vi "interface alive.vi"(8 "error in (no error)":errorcluster, 11 "output_actor in":refnum<class "Output Actor.lvclass">) -> (0 "error out":errorcluster, 2 "alive":bool, 3 "output_actor out":refnum<class "Output Actor.lvclass">)   [LabVIEW 2015, in "Output Actor.lvclass"]
uses:
  Output Actor.lvclass
  Output Actor.lvclass/Output Actor.ctl
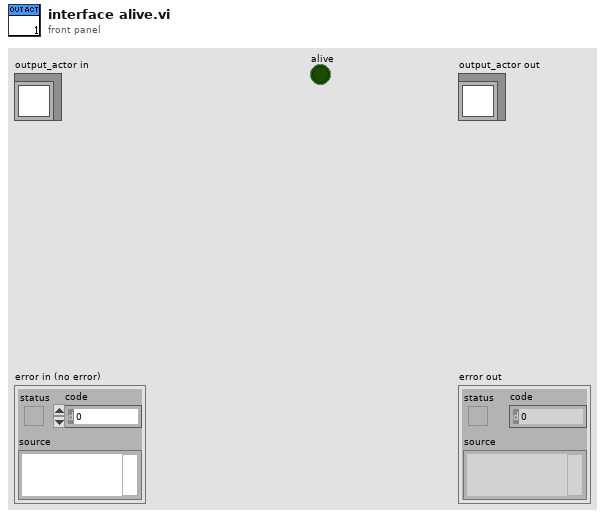
[diagram p1: front panel]
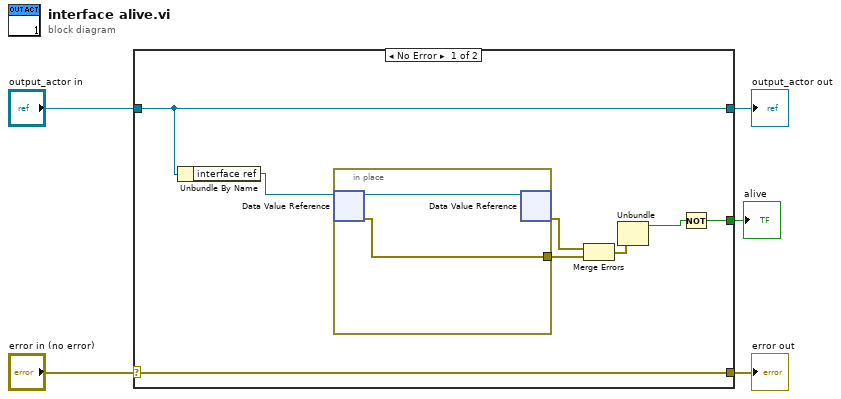
[diagram p0: block diagram]
diagram:
  n1 = case shown="No Error" "error in (no error)" {
    selector: "error in (no error)" -> [w13 w17]
    tunnel: [w13 w17] -> w4
    tunnel: [w7 w16] -> w2
    tunnel: "output_actor in" -> [w7 w16]
    tunnel: [w6 _] -> w1
    frame No Error {
      n2 = Unbundle By Name(w7) -> ("interface ref"=w12:refnum<data-value>)
      n3 = in-place {
        in-place-border: [w14] -> w10
        n4 = in-place-dvr #1(w12) -> (w15:refnum<class "Output Actor Interface.lvclass">, w14:errorcluster)
        n5 = in-place-dvr #1(w15) -> (w11:errorcluster)  [unwired: 1 out]
      }
      n6 = Merge Errors(w11, w10) -> (w9:errorcluster)
      n7 = Unbundle(w9) -> ("status"=w8:bool)  [unwired: 2 out]
      n8 = Not(x=w8) -> (.not. x?=w6:bool)
    }
    frame Error {
    }
  }
  "error out" <- w4
  "output_actor out" <- w2
  "alive" <- w1
